vi "BuildChannelListFromChannels.vi"(0 "Channels (A:B:C:D...) (In)":string, 5 "Channel Names (In)":string[](array[string])) -> (4 "Channel List (Out)":string[](array[string]), 6 "Channels (Out)":i32[](array[numeric]))   [LabVIEW 2015]
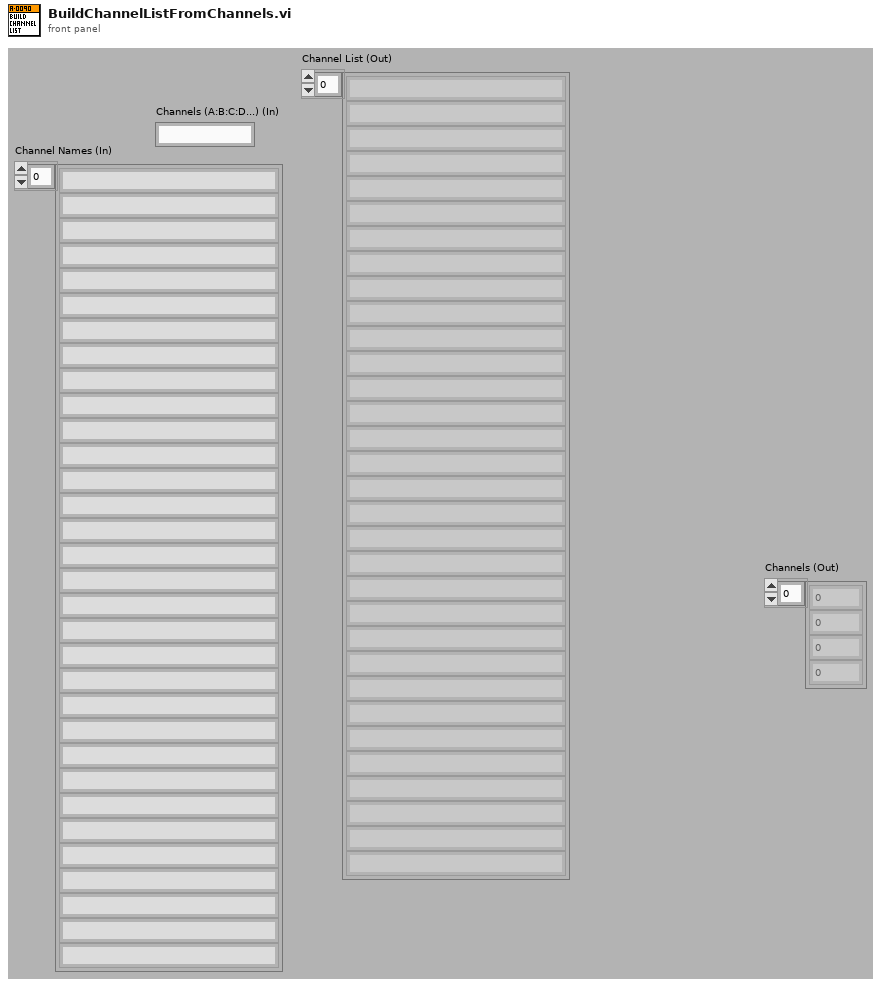
[diagram p1: front panel]
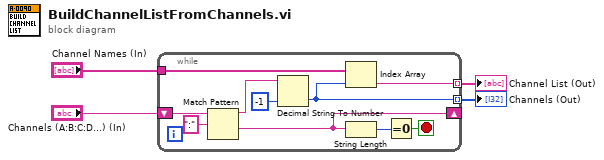
[diagram p0: block diagram]
diagram:
  n1 = while {
    shift-right: [w12] -> _
    shift-left: "Channels (A:B:C:D...) (In)" -> [w14]
    tunnel: "Channel Names (In)" -> [w8]
    tunnel: [w6] -> w2 mode=indexing
    tunnel: [w5] -> w1 mode=indexing
    stop <- w10 stop-if-true
    n2 = Match Pattern(string=w14, regular expression=":") -> (before substring=w9:string, after substring=w12:string)  [unwired: 1 in, 2 out]
    n3 = Decimal String To Number(string=w9, default (0L)=-1 ("default (0 I32)")) -> (number=w5:i32)  [unwired: 1 in, 1 out]
    n4 = Index Array(array=w8, index=w5) -> (element=w6:string)
    n5 = String Length(string=w12) -> (length=w11:i32)
    n6 = Equal To 0?(x=w11) -> (x = 0?=w10:bool)
  }
  "Channel List (Out)" <- w2
  "Channels (Out)" <- w1
